vi "Update Plugin Tree with New Script Value.vi"(8 "error in (no error)":errorcluster, 9 "New Script":string, 10 "OrigPluginTreeTags":string[](array[string]), 11 "TreeControl in":refnum<vi>) -> (0 "error out":errorcluster, 3 "Tree ref out":refnum<vi>)   [LabVIEW 2018]
uses:
  Controls/Plugins Tree Item Type.ctl
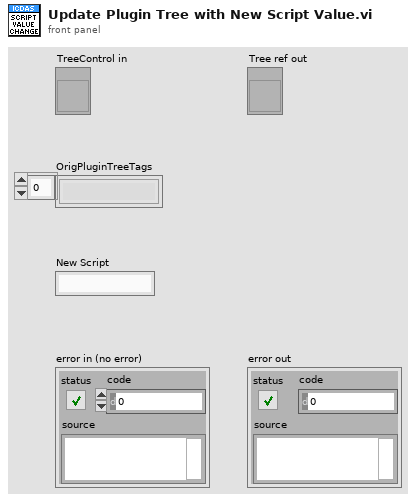
[diagram p1: front panel]
types:
  T1 = typedef "Plugins Tree Item Type.ctl" = enum16{"Plugin", "Instrument", "INI File", "INI Script"}
  T2 = typedef "Plugin Tree Tag.ctl" = cluster{"ItemType":T1, "Name":string, "Path":path, "Script":string[]}
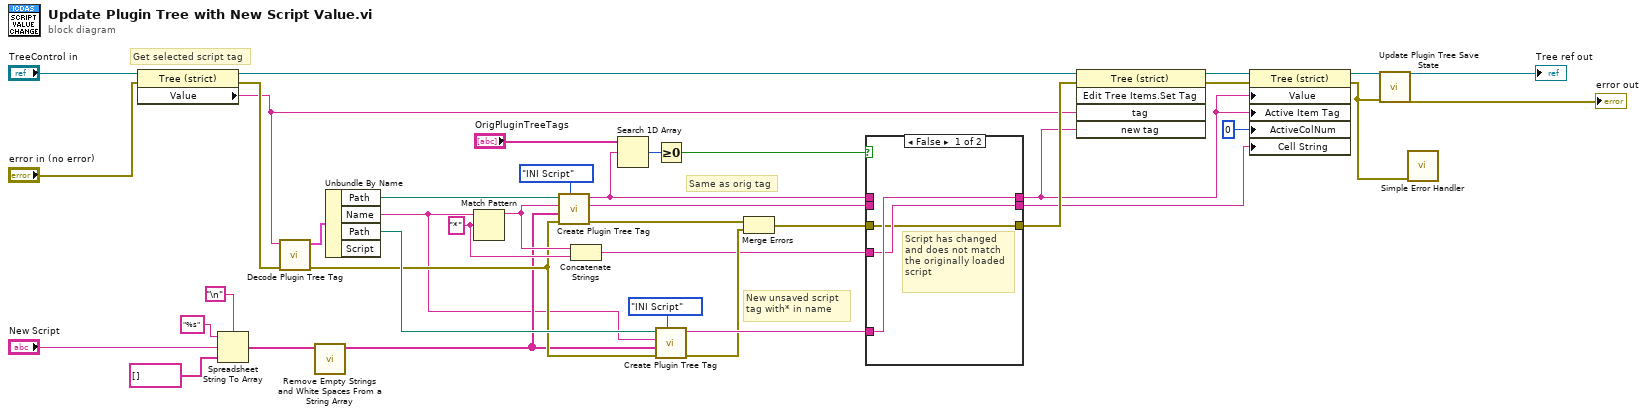
[diagram p0: block diagram]
diagram:
  w37 = "*" ("regular expression")
  # "New unsaved script\ntag with* in name"
  # "Same as orig tag"
  # "Get selected script tag"
  n1 = property class="Tree (strict)"(reference="TreeControl in", error in="error in (no error)") -> (reference out=w17:refnum<vi>, error out=w25:errorcluster, "Value"=w10:string)
  n2 = Spreadsheet String To Array(delimiter (Tab)="\n", format string="%s", spreadsheet string="New Script", array type (2D Dbl)=string[] [] ("Script")) -> (array=w6:string[])
  n3 = call "Decode Plugin Tree Tag.vi"("error in (no error)"=w25, "Tag"=w10) -> ("error out"=w24:errorcluster, "Plugin Tree Tag"=w28:T2)  [unwired: 8 in]
  n4 = call "Remove Empty Strings and White Spaces From a String Array.vi"("Array in"=w6) -> ("Array out"=w8:string[])  [unwired: 10 in]
  n5 = Unbundle By Name(w28) -> ("Path"=w29:path, "Name"=w3:string, "Path"=w38:path)  [unwired: 1 out]
  n6 = Match Pattern(string=w3, regular expression=w37) -> (before substring=w36:string)  [unwired: 1 in, 3 out]
  n7 = call "Create Plugin Tree Tag.vi"("ItemType"=Plugins_Tree_Item_Type."INI Script", "error in (no error)"=w24, "Script"=w8, "Name"=w36, "VISA Resource"=w29) -> ("error out"=w20:errorcluster, "Name out"=w23:string, "Tag"=w21:string)  [unwired: 4 in]
  n8 = Concatenate Strings(w36, w37) -> (w2:string)
  n9 = Search 1D Array(1D array="OrigPluginTreeTags", element=w21) -> (index of element=w35:i32)  [unwired: 1 in]
  n10 = Greater Or Equal To 0?(x=w35) -> (x >= 0?=w7:bool)
  n11 = call "Create Plugin Tree Tag.vi"("ItemType"=Plugins_Tree_Item_Type."INI Script", "error in (no error)"=w24, "Script"=w8, "Name"=w3, "VISA Resource"=w38) -> ("error out"=w18:errorcluster, "Tag"=w22:string)  [unwired: 4 in, 1 out]
  n12 = Merge Errors(w20, w18) -> (w19:errorcluster)
  n13 = case shown="False" w7 {
    tunnel: w19 -> [w41 w44]
    tunnel: w23 -> [_ w45]
    tunnel: w2 -> [w42 _]
    tunnel: w22 -> [w43 _]
    tunnel: w21 -> [_ w46]
    tunnel: [w43 w46] -> w1
    tunnel: [w42 w45] -> w12
    tunnel: [w41 w44] -> w16
    frame False {
      # "Script has changed\nand does not match\nthe originally loaded\nscript"
    }
    frame True {
      # "Script has changed\nand matches\nthe originally loaded\nscript"
    }
  }
  n14 = invoke class="Tree (strict)" method="Edit Tree Items.Set Tag"(reference=w17, error in=w16, "tag"=w10, "new tag"=w1) -> (reference out=w15:refnum<vi>, error out=w14:errorcluster)  [unwired: 1 in, 3 out]
  n15 = property class="Tree (strict)"(reference=w15, error in=w14, "Value"=w1, "Active Item Tag"=w1, "ActiveColNum"=0 ("Active Cell:Active Column Number"), "Cell String"=w12) -> (reference out=w11:refnum<vi>, error out=w9:errorcluster)
  n16 = call "Update Plugin Tree Save State.vi"("error in (no error)"=w9, "TreeControl in"=w11) -> ("error out"=→"error out":errorcluster, "TreeControl out"=→"Tree ref out":refnum<vi>)  [unwired: 8 in]
  n17 = call <vilib>:"Simple Error Handler.vi"("error in (no error)"=w9) -> ()  [unwired: 4 in, 5 out]
